vi "Set Signal Polarity.vi"(8 "error in (no error)":errorcluster {"code" format="%.0x"}, 9 "Polarity (T:POS)":bool=TRUE, 10 "Signal Connector (0:TRIGGER IN)":T1(ring), 11 "VISA Resource Name":refnum<visa-resource-name>) -> (0 "error out":errorcluster {"code" format="%.0x"}, 3 "VISA Resource Name Out":refnum<visa-resource-name>)   [LabVIEW 2012, in "Agilent ESG Series.lvlib"]
doc: "This VI is set the polarity of various signal outputs and inputs."
uses:
  <instrlib>/Agilent ESG Series/Agilent ESG Series.lvlib
panel:
  # "POS"
  # "NEG"
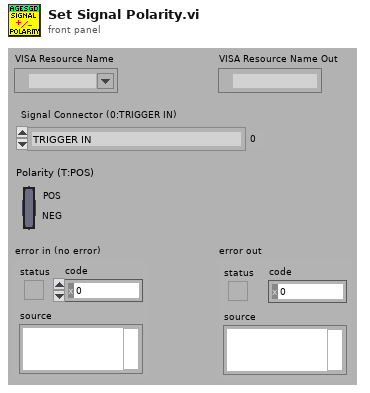
[diagram p1: front panel]
types:
  T1 = enum16{"TRIGGER IN", "DATA IN", "DATA CLOCK INPUT", "SYMBOL SYNC INPUT", "BURST GATE IN", "PATTERN TRIGGER IN", "TRIGGER OUT", "DATA OUT", "DATA CLOCK OUT", "SYMBOL SYNC OUT", "EVENT 1", "EVENT 2", "EVENT 3", "EVENT 4"}
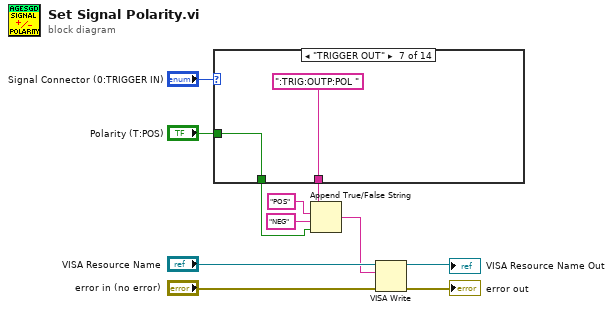
[diagram p0: block diagram]
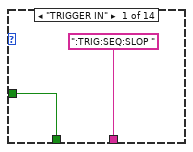
[diagram p2: hidden frame]
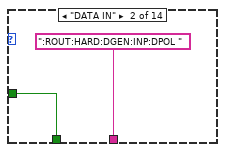
[diagram p3: hidden frame]
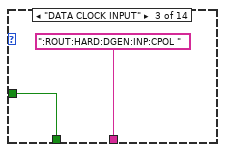
[diagram p4: hidden frame]
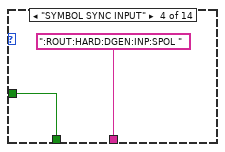
[diagram p5: hidden frame]
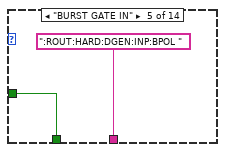
[diagram p6: hidden frame]
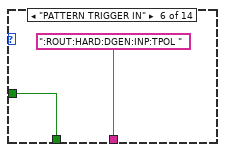
[diagram p7: hidden frame]
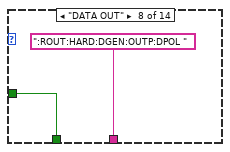
[diagram p8: hidden frame]
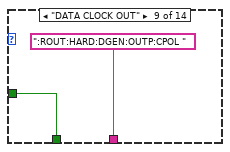
[diagram p9: hidden frame]
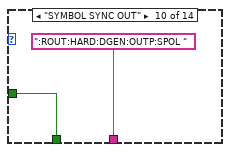
[diagram p10: hidden frame]
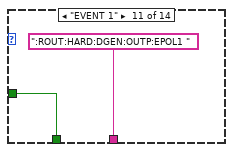
[diagram p11: hidden frame]
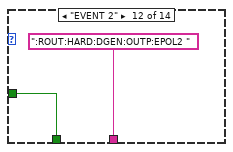
[diagram p12: hidden frame]
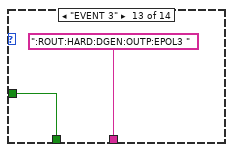
[diagram p13: hidden frame]
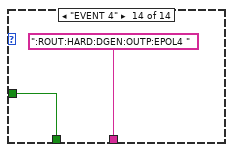
[diagram p14: hidden frame]
diagram:
  n1 = case shown="\"TRIGGER OUT\"" "Signal Connector (0:TRIGGER IN)" {
    tunnel: [":TRIG:SEQ:SLOP " ":ROUT:HARD:DGEN:INP:DPOL " ":ROUT:HARD:DGEN:INP:CPOL " ":ROUT:HARD:DGEN:INP:SPOL " ":ROUT:HARD:DGEN:INP:BPOL " ":ROUT:HARD:DGEN:INP:TPOL " ":TRIG:OUTP:POL " ":ROUT:HARD:DGEN:OUTP:DPOL " ":ROUT:HARD:DGEN:OUTP:CPOL " ":ROUT:HARD:DGEN:OUTP:SPOL " ":ROUT:HARD:DGEN:OUTP:EPOL1 " ":ROUT:HARD:DGEN:OUTP:EPOL2 " ":ROUT:HARD:DGEN:OUTP:EPOL3 " ":ROUT:HARD:DGEN:OUTP:EPOL4 "] -> w3
    tunnel: [w12 w14 w16 w18 w20 w22 w24 w26 w28 w30 w32 w34 w36 w38] -> w2
    tunnel: "Polarity (T:POS)" -> [w12 w14 w16 w18 w20 w22 w24 w26 w28 w30 w32 w34 w36 w38]
    frame "TRIGGER IN" {
    }
    frame "DATA IN" {
    }
    frame "DATA CLOCK INPUT" {
    }
    frame "SYMBOL SYNC INPUT" {
    }
    frame "BURST GATE IN" {
    }
    frame "PATTERN TRIGGER IN" {
    }
    frame "TRIGGER OUT" {
    }
    frame "DATA OUT" {
    }
    frame "DATA CLOCK OUT" {
    }
    frame "SYMBOL SYNC OUT" {
    }
    frame "EVENT 1" {
    }
    frame "EVENT 2" {
    }
    frame "EVENT 3" {
    }
    frame "EVENT 4" {
    }
  }
  n2 = Append True/False String(1:w2, 2:"NEG" ("false string"), 3:"POS" ("true string"), 4:w3) -> (0:w6:string)
  n3 = VISA Write(VISA resource name="VISA Resource Name", write buffer=w6, error in (no error)="error in (no error)") -> (VISA resource name out=→"VISA Resource Name Out":refnum<visa-resource-name>, error out=→"error out":errorcluster)  [unwired: 1 out]
